vi "FahrenheitToCelciusConverter.vi"() -> ()   [LabVIEW 2024]
panel:
  in  "stop":bool
  out "Thermometer (C)":dbl
  in  "Temperature (F)":dbl
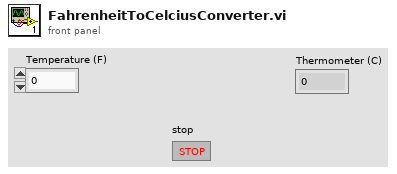
[diagram p1: front panel]
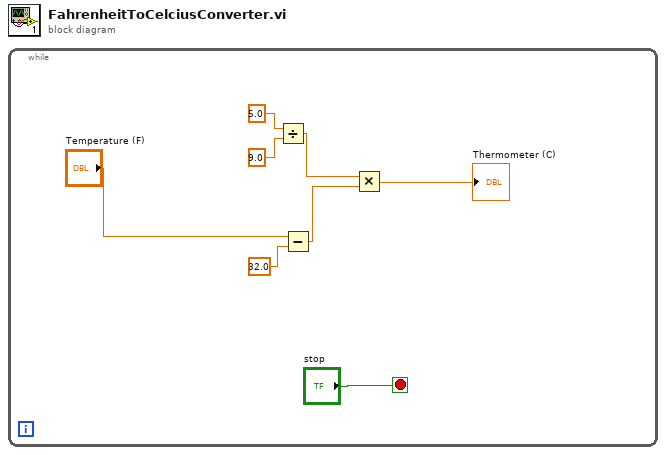
[diagram p0: block diagram]
diagram:
  n1 = while {
    stop <- "stop" stop-if-true
    n2 = Divide(x=5.0, y=9.0) -> (x/y=w4:dbl)
    n3 = Subtract(x="Temperature (F)", y=32.0) -> (x-y=w3:dbl)
    n4 = Multiply(x=w4, y=w3) -> (x*y=→"Thermometer (C)":dbl)
  }
